vi "Command Package.vi"(0 "UART_Command":T1, 1 "Channel Number":u8, 5 "Cmd_data":u16) -> (4 "Cmd_package":u32)   [LabVIEW 2012, in "UART_Host_Driver.lvlib" / "UART Driver.lvclass"]
uses:
  UART Driver.lvclass
  FPGA/UART/UART_Command.ctl
  FPGA/UART/UART_Firmware.lvlib
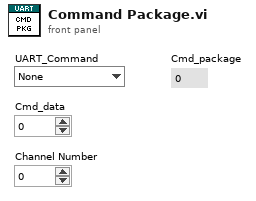
[diagram p1: front panel]
types:
  T1 = typedef "UART_Firmware.lvlib/UART_Command.ctl" = enum8{"None", "Tx", "SetBaud_High", "SetBaud_Low", "SetCharLength", "SetParity", "SetStopBits", "SetSpacing_High", "SetSpacing_Low"}
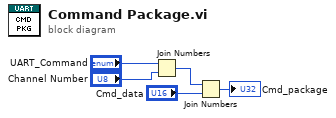
[diagram p0: block diagram]
diagram:
  n1 = Join Numbers(hi="UART_Command", lo="Channel Number") -> ((hi.lo)=w4:u16)
  n2 = Join Numbers(hi=w4, lo="Cmd_data") -> ((hi.lo)=→"Cmd_package":u32)
